vi "Set Param.vi"(8 "error in (no error)":errorcluster, 11 "socket PUB in":refnum<class "socket PUB.lvclass">) -> (0 "error out":errorcluster, 3 "socket PUB out":refnum<class "socket PUB.lvclass">)   [LabVIEW 2018, in "socket PUB.lvclass"]
uses:
  socket PUB.lvclass
  <vilib>/addons/zeromq/socket_type.ctl
  <vilib>/addons/zeromq/zeromq.lvlib
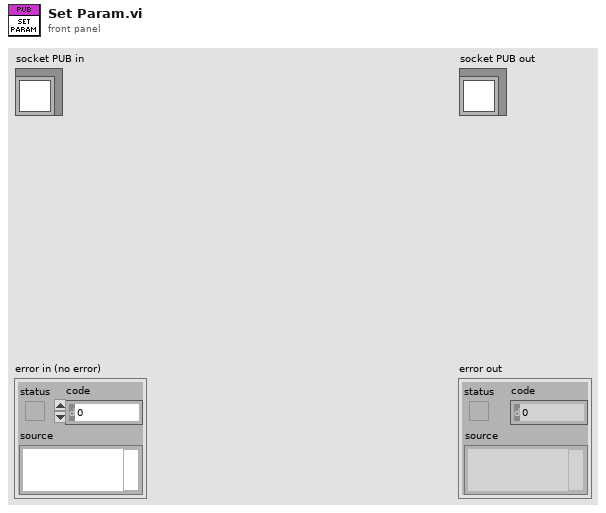
[diagram p1: front panel]
types:
  T1 = typedef "zeromq.lvlib/socket_type.ctl" = enum8{"ZMQ_PAIR", "ZMQ_PUB", "ZMQ_SUB", "ZMQ_REQ", "ZMQ_REP", "ZMQ_DEALER", "ZMQ_ROUTER", "ZMQ_PULL", "ZMQ_PUSH", "ZMQ_XPUB", "ZMQ_XSUB", "ZMQ_STREAM", "ZMQ_SERVER", "ZMQ_CLIENT", "ZMQ_RADIO", "ZMQ_DISH", "ZMQ_GATHER", "ZMQ_SCATTER", "ZMQ_DGRAM"}
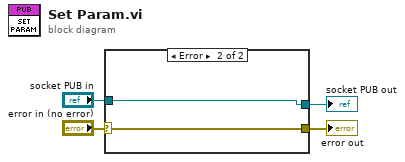
[diagram p0: block diagram]
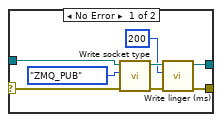
[diagram p2: hidden frame]
diagram:
  n1 = case shown="Error" "error in (no error)" {
    selector: "error in (no error)" -> [w10 w13]
    tunnel: "socket PUB in" -> [w9 w14]
    tunnel: [w6 w14] -> w2
    tunnel: [w5 w13] -> w1
    frame No Error {
      n2 = call-dynamic "Write socket type.vi"("error in (no error)"=w10, "Socket type"=socket_type."ZMQ_PUB", "Socket in"=w9) -> ("error out"=w11:errorcluster, "Socket out"=w12:refnum<class "socket PUB.lvclass">)  [unwired: 7 in]
      n3 = call-dynamic "Write linger (ms).vi"("error in (no error)"=w11, "linger (ms)"=200, "Socket in"=w12) -> ("error out"=w5:errorcluster, "Socket out"=w6:refnum<class "socket PUB.lvclass">)  [unwired: 7 in]
    }
    frame Error {
    }
  }
  "error out" <- w1
  "socket PUB out" <- w2
